vi "Sample MICS Connection Attempts.vi"(4 "Number of \"Open Session\" Retry Attempts (3)":i32=3, 6 "2.45 GHz Wake-Up Power":i8(ring)=6 items=["-29"=-29, "-4"=-4, "-2"=-2, "0"=0, "2"=2, "4"=4, "6"=6, "8"=8, "10"=10, "12"=12, "14"=14, "16"=16, "18"=18, "20"=20, "22"=22, "24"=24, "26"=26, "27"=27], 7 "400 MHz MICS Power Setting":u8=22 format="%02x", 8 "error in":errorcluster, 9 "Attenuation dB":dbl, 10 "Samples (1)":i32=1, 11 "MICS Resource Name":refnum<visa-resource-name>) -> (0 "error out":errorcluster, 1 "Number Successful":i16, 2 "Percent Successful":dbl, 3 "MICS Resource Name out":refnum<visa-resource-name>)   [LabVIEW 2010]
doc: "Author: Nick Stevens (ERIK JAGGER EDITS)\n\nSamples N connection attempts with the configured MICS ID, returning the percentage of successful attempts."
panel:
  out "Abort Elapsed":u32[](array[numeric])
  out "Start Elapsed":u32[](array[numeric])
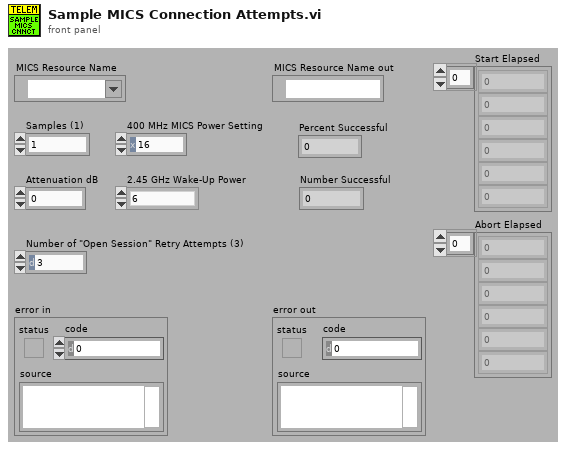
[diagram p1: front panel]
types:
  T1 = enum16{"Get Device Type", "Get Device Name", "Get Device Version", "Get Device Error"}
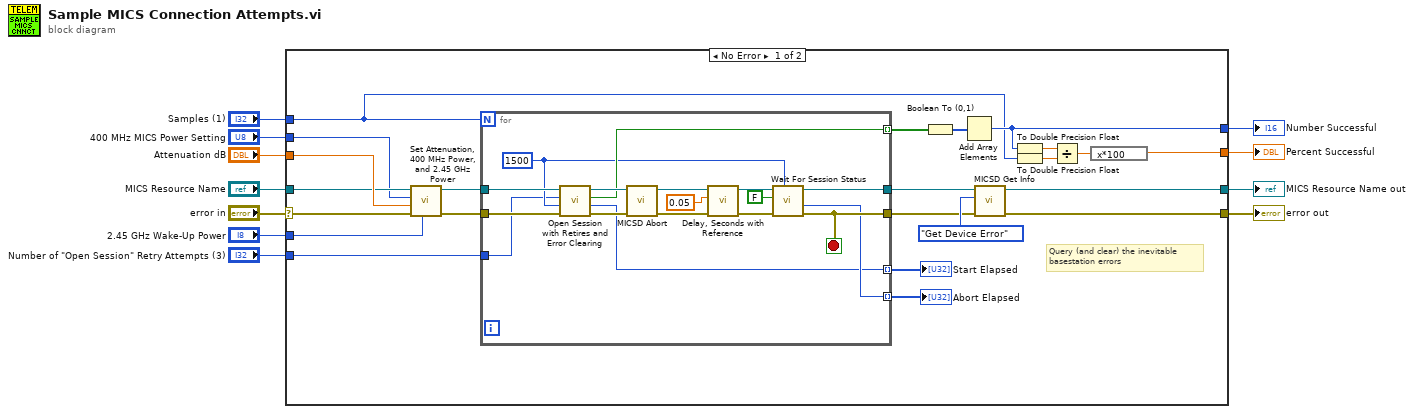
[diagram p0: block diagram]
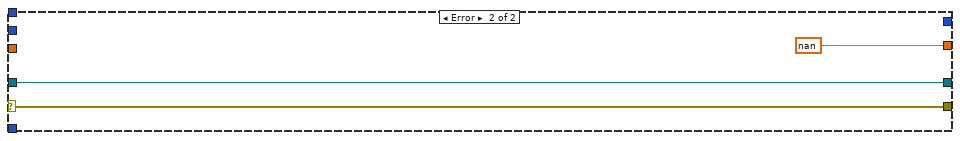
[diagram p2: hidden frame]
diagram:
  n1 = case shown="No Error" "error in" {
    selector: "error in" -> [w18 w53]
    tunnel: [w34 nan] -> w11
    tunnel: [w32 _] -> w10
    tunnel: "Samples (1)" -> [w31 _]
    tunnel: "MICS Resource Name" -> [w16 w54]
    tunnel: [w22 w53] -> w7
    tunnel: [w23 w54] -> w6
    tunnel: "Attenuation dB" -> [w19 _]
    tunnel: "400 MHz MICS Power Setting" -> [w15 _]
    tunnel: "2.45 GHz Wake-Up Power" -> [w13 _]
    tunnel: "Number of \"Open Session\" Retry Attempts (3)" -> [w12 _]
    frame No Error {
      # "Query (and clear) the inevitable\nbasestation errors"
      n2 = call "Set Attenuation, 400 MHz Power, and 2.45 GHz Power.vi"("2.45 GHz Wake-Up Power (6)"=w13, "error in"=w18, "Attenuation dB (0)"=w19, "400 MHz MICS Power Setting (0x16)"=w15, "VISA Resource Name"=w16) -> ("error out"=w17:errorcluster, "dup VISA Resource Name"=w14:refnum<visa-resource-name>)  [unwired: 5 in]
      n3 = for {
        N: w31 -> [_]
        tunnel: [w50] -> w25
        tunnel: [w49] -> w24
        tunnel: [w42] -> w29 mode=indexing
        tunnel: [w43] -> w21 mode=indexing
        tunnel: [w48] -> w20 mode=indexing
        tunnel: w17 -> [w47]
        tunnel: w14 -> [w45]
        tunnel: w12 -> [w40]
        stop <- w49 stop-if-true
        w41 = u32 1500 ("Timeout (3000 ms)")
        n4 = call "Open Session with Retires and Error Clearing.vi"("error in"=w47, "\"Wait for Session\" Timeout (3000 ms)"=w41, "Number of \"Open Session\" Retry Attempts (3)"=w40, "VISA Resource Name"=w45) -> ("error out"=w46:errorcluster, "Elapsed Time (ms)"=w43:u32, "IN_SESSION"=w42:bool, "dup VISA Resource Name"=w44:refnum<visa-resource-name>)  [unwired: 4 in]
        n5 = call "MICSD Abort.vi"("error in (no error)"=w46, "VISA Resource Name"=w44) -> ("error out"=w37:errorcluster, "dup VISA Resource Name"=w39:refnum<visa-resource-name>)  [unwired: 8 in]
        n6 = call "Delay, Seconds with Reference.vi"("error in"=w37, "delay"=dbl[unit] 0.05, "VISA resource"=w39) -> ("error out"=w36:errorcluster, "VISA resource dup"=w38:refnum<visa-resource-name>)  [unwired: 3 in, 1 out]
        n7 = call "Wait For Session Status.vi"("Timeout (3000 ms)"=w41, "error in (no error)"=w36, "IN_SESSION State (T)"=FALSE, "VISA Resource Name"=w38) -> ("error out"=w49:errorcluster, "Elapsed Time (ms)"=w48:u32, "dup VISA Resource Name"=w50:refnum<visa-resource-name>)  [unwired: 4 in, 1 out]
      }
      "Start Elapsed" <- w21
      "Abort Elapsed" <- w20
      n8 = Boolean To (0,1)(Boolean=w29) -> (0, 1=w30:i16[])
      n9 = Add Array Elements(numeric array=w30) -> (sum=w32:i16)
      n10 = call "MICSD Get Info.vi"("error in (no error)"=w24, "Command"=T1."Get Device Error", "VISA Resource Name"=w25) -> ("error out"=w22:errorcluster, "dup VISA Resource Name"=w23:refnum<visa-resource-name>)  [unwired: 6 in, 1 out]
      n11 = To Double Precision Float(number=w32) -> (double precision float=w28:dbl)
      n12 = To Double Precision Float(number=w31) -> (double precision float=w27:dbl)
      n13 = Divide(x=w28, y=w27) -> (x/y=w33:dbl)
      n14 = expression code="x*100"(w33) -> (w34:dbl)
    }
    frame Error {
    }
  }
  "Percent Successful" <- w11
  "error out" <- w7
  "MICS Resource Name out" <- w6
  "Number Successful" <- w10
